vi "Laser_Control_3D.vi"() -> ()   [LabVIEW 2022 SP3]
uses:
  ADAM Client/Sub VIs/ADAM Controls/Update_scan_value.ctl
  Fibre_Flow_Mode.ctl
panel:
  in  "BSA IP Number":string="10.10.100.130"
  in  "Laser3":string="LAN10.10.100.127"
  in  "Laser2":string="LAN10.10.100.121"
  in  "Laser1":string="LAN10.10.100.120"
  out "error out  BSA":errorcluster
  in  "Power (mW) 3":dbl
  out "Status 3":string[](array[string])
  in  "BSALaserCtrl.IBSALaser 4":refnum<k7>
  out "GetMaxPower (mW) 3":dbl
  in  "Mode 3":T1
  out "error out 3":errorcluster
  out "Loop No 3":i32
  in  "Power (mW) 2":dbl
  out "Status 2":string[](array[string])
  in  "BSALaserCtrl.IBSALaser 3":refnum<k7>
  out "GetMaxPower (mW) 2":dbl
  in  "Mode 2":T1
  out "error out 2":errorcluster
  out "Loop No 2":i32
  out "GetMaxPower (mW)":dbl
  in  "stop":bool
  out "Loop No":i32
  in  "Power (mW)":dbl
  in  "Mode":T1
  out "error out":errorcluster
  in  "BSALaserCtrl.IBSALaser 2":refnum<k7>
  out "Status":string[](array[string])
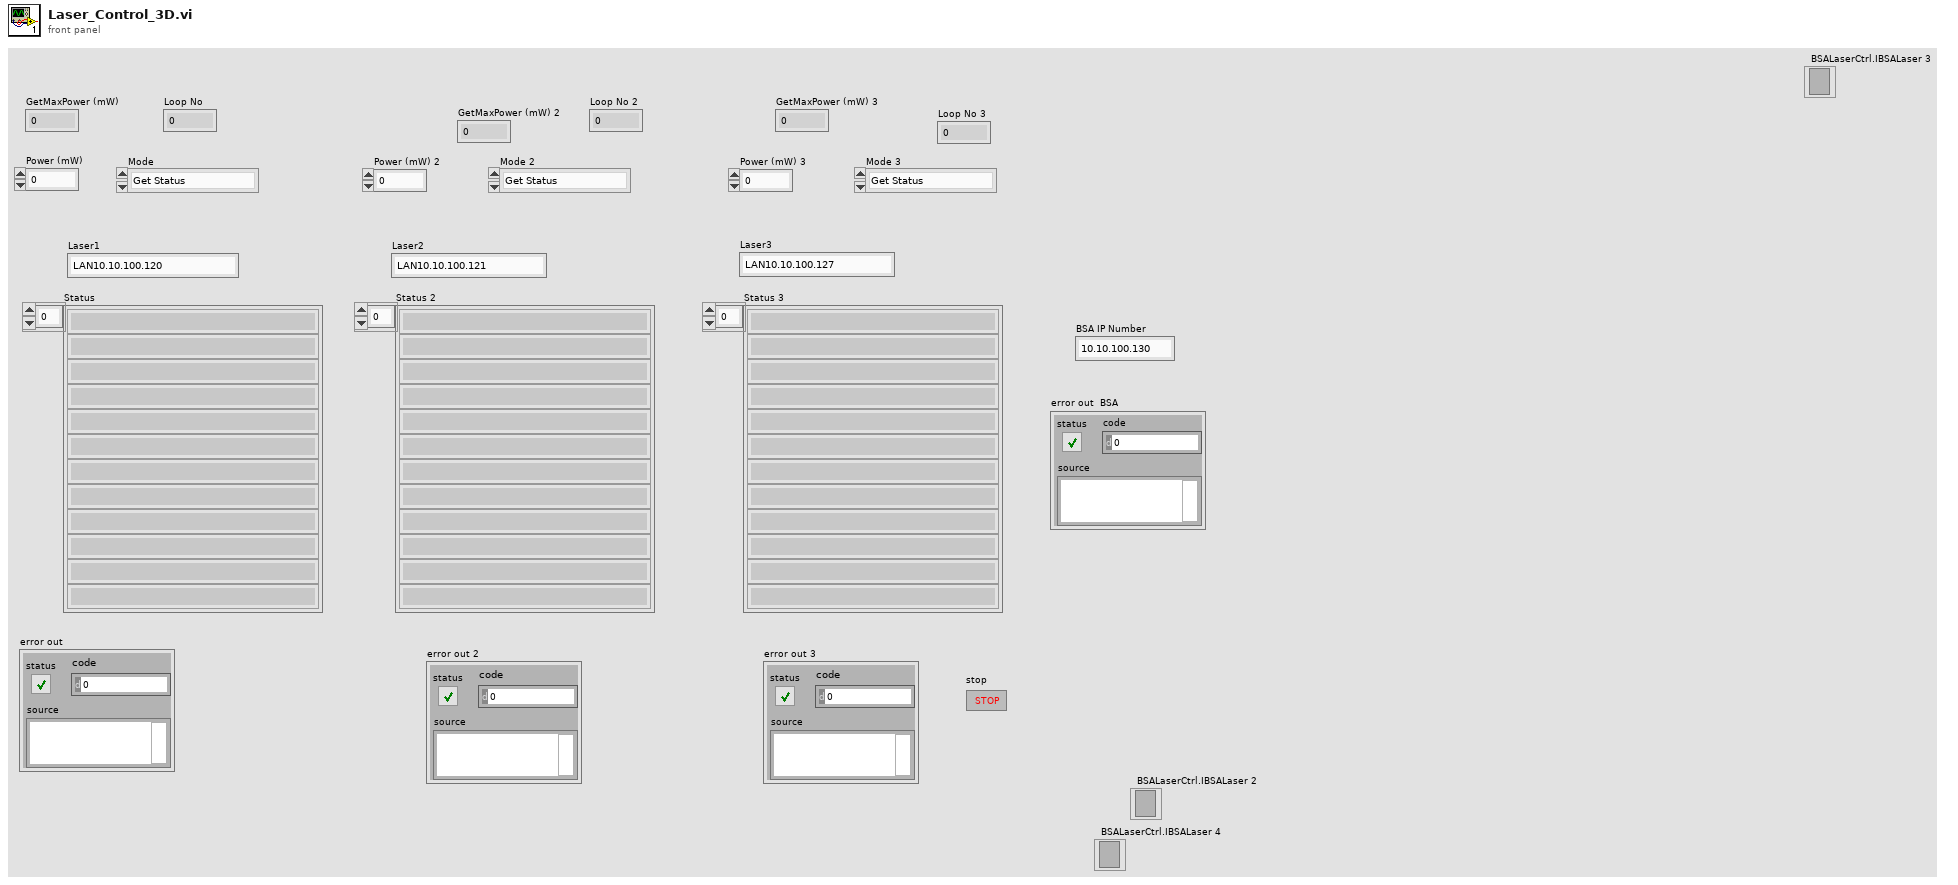
[diagram p1: front panel]
types:
  T1 = typedef "Fibre_Flow_Mode.ctl" = enum16{"Get Status", "Set Power", "Turn Laser On", "Turn Laser Off", "Shutter Open", "Shutter Closed", "Attenuated", "Disconnect"}
  T2 = typedef "Update_scan_value.ctl" = cluster{"Channel Name":string, "New Value":dbl, "!Auto_Off":bool}
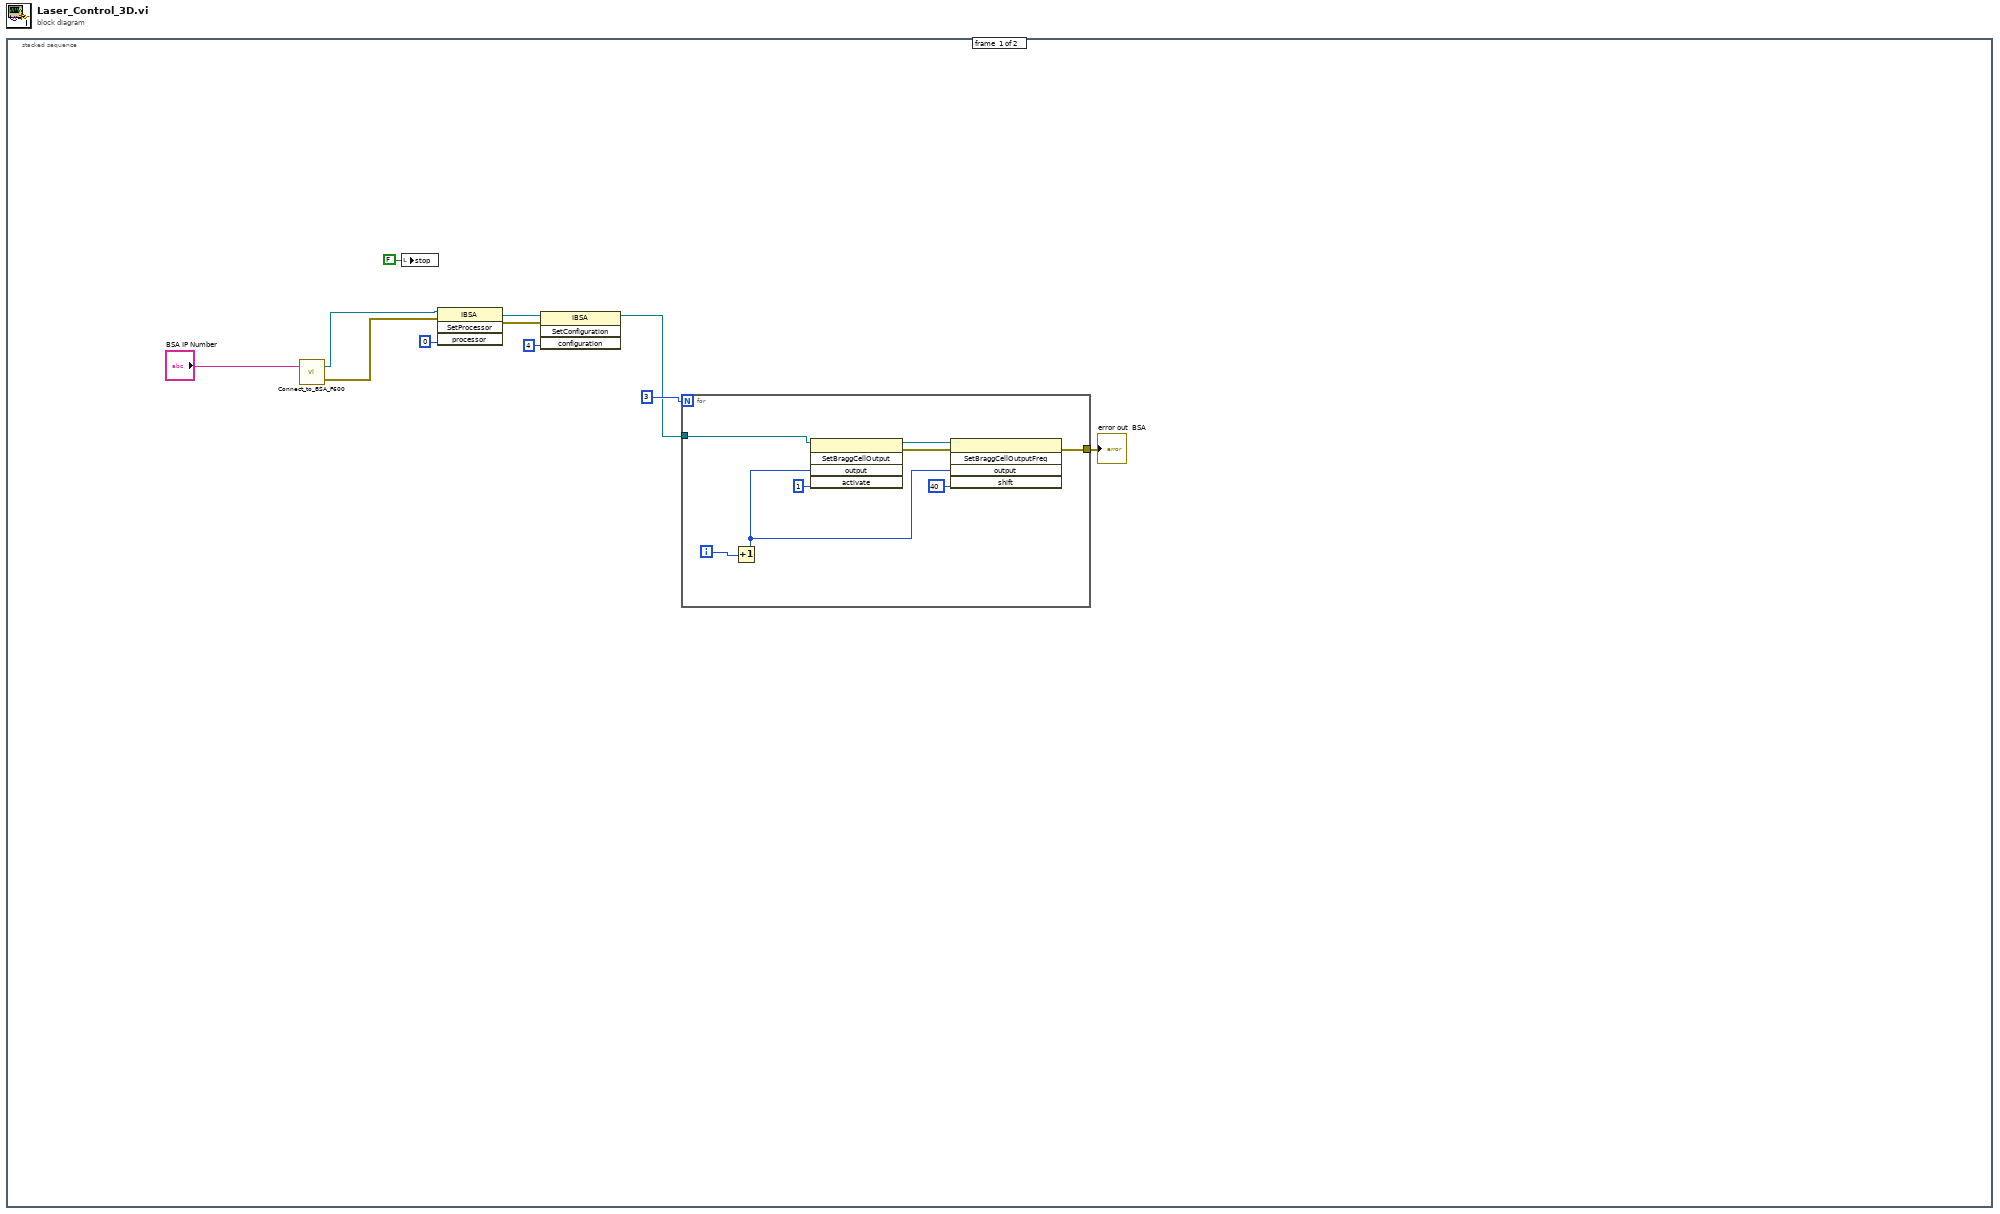
[diagram p0: block diagram]
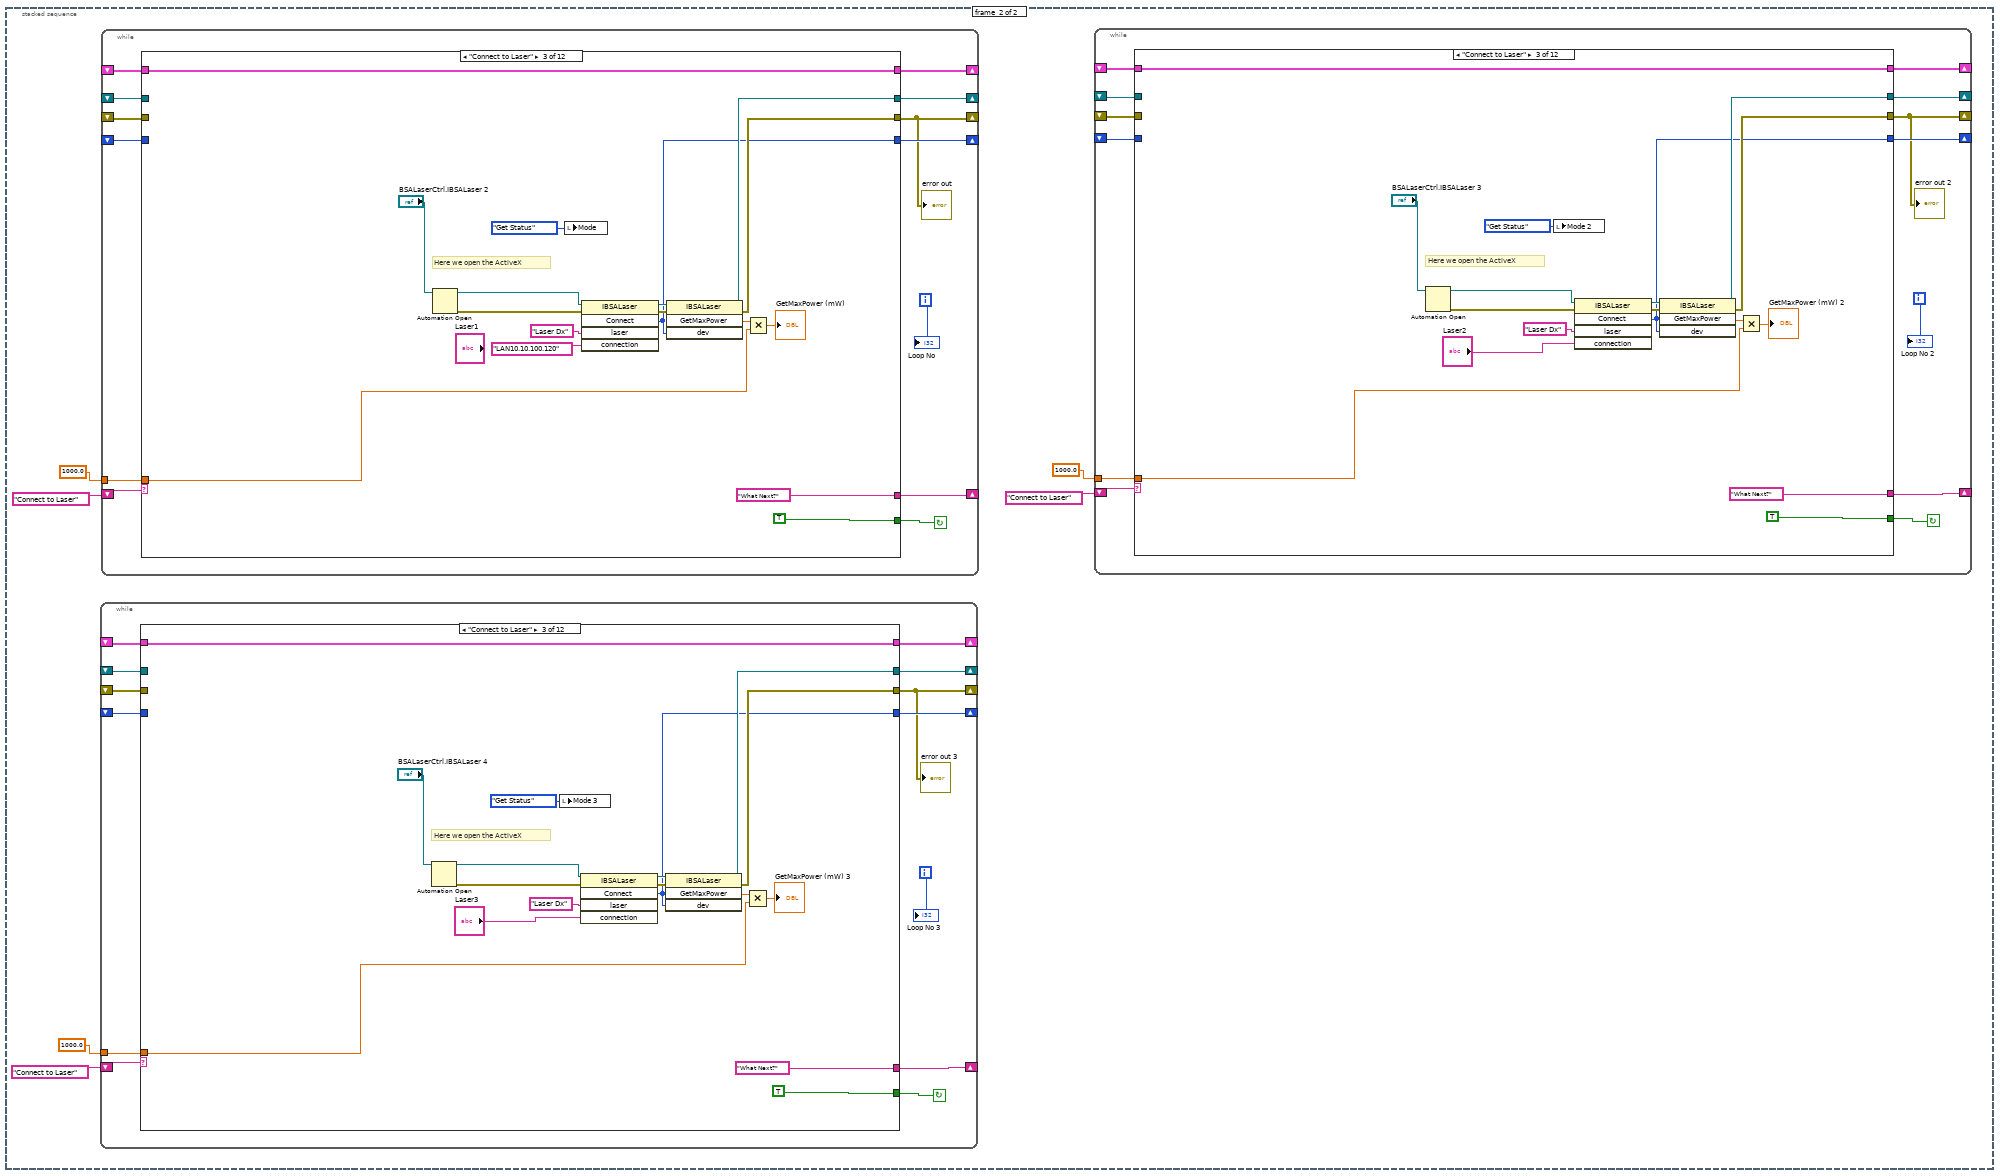
[diagram p2: hidden frame]
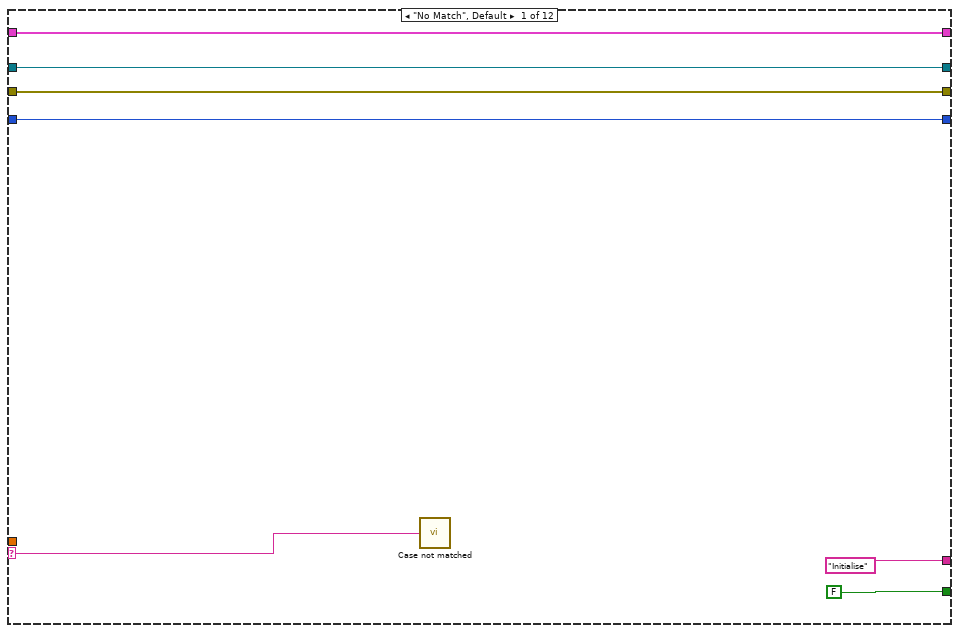
[diagram p3: hidden frame]
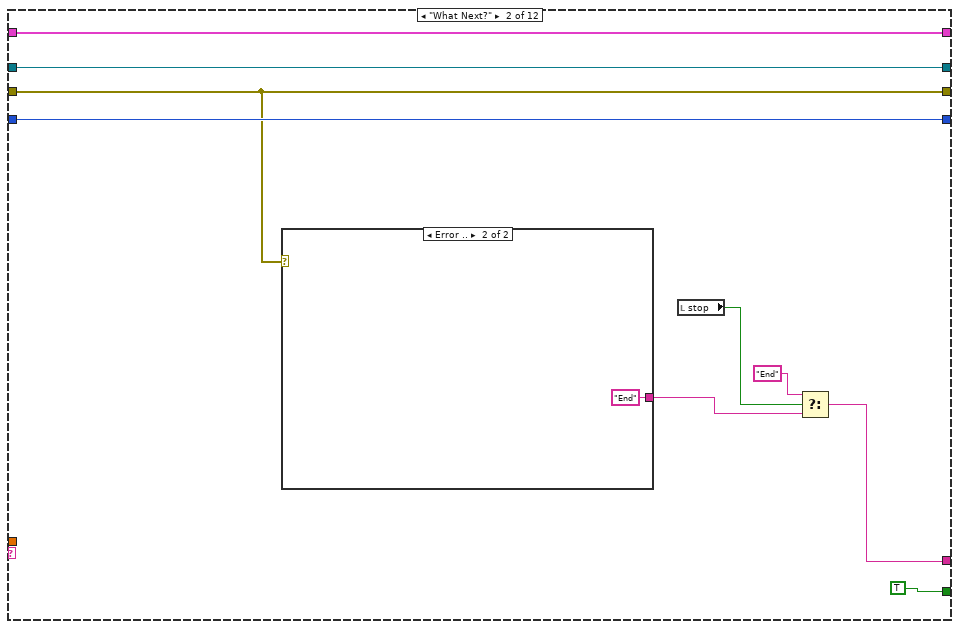
[diagram p4: hidden frame]
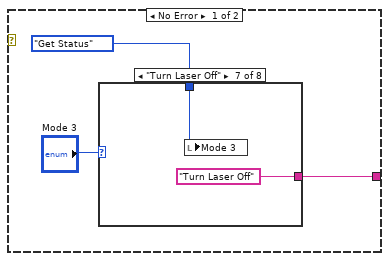
[diagram p5: hidden frame]
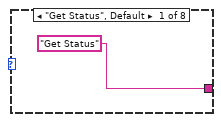
[diagram p6: hidden frame]
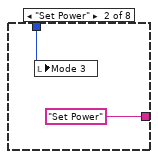
[diagram p7: hidden frame]
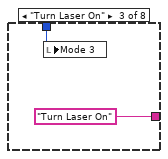
[diagram p8: hidden frame]
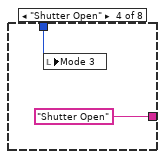
[diagram p9: hidden frame]
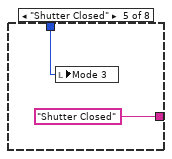
[diagram p10: hidden frame]
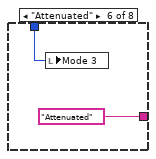
[diagram p11: hidden frame]
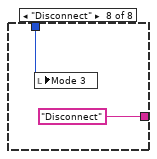
[diagram p12: hidden frame]
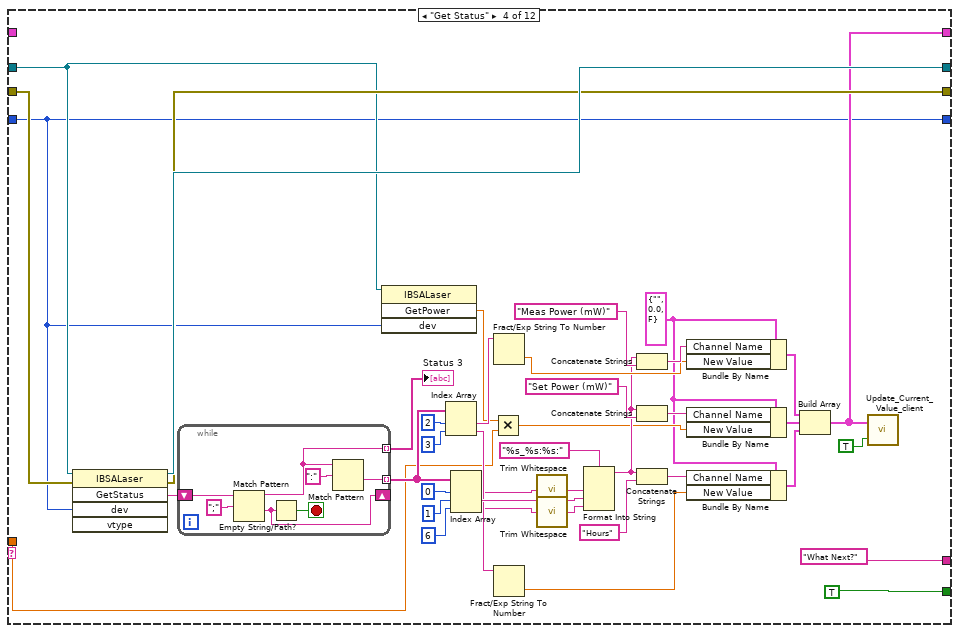
[diagram p13: hidden frame]
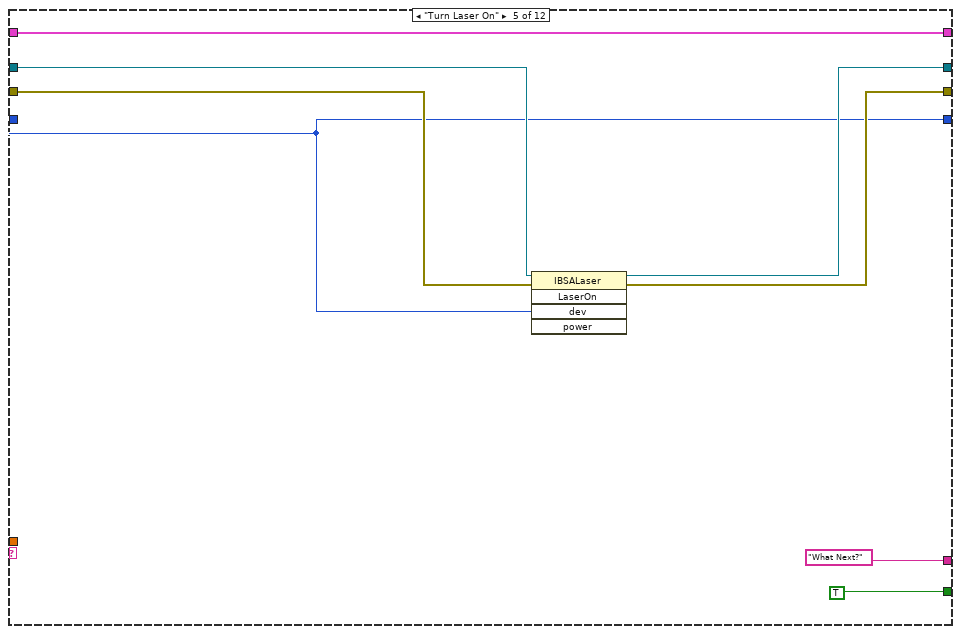
[diagram p14: hidden frame]
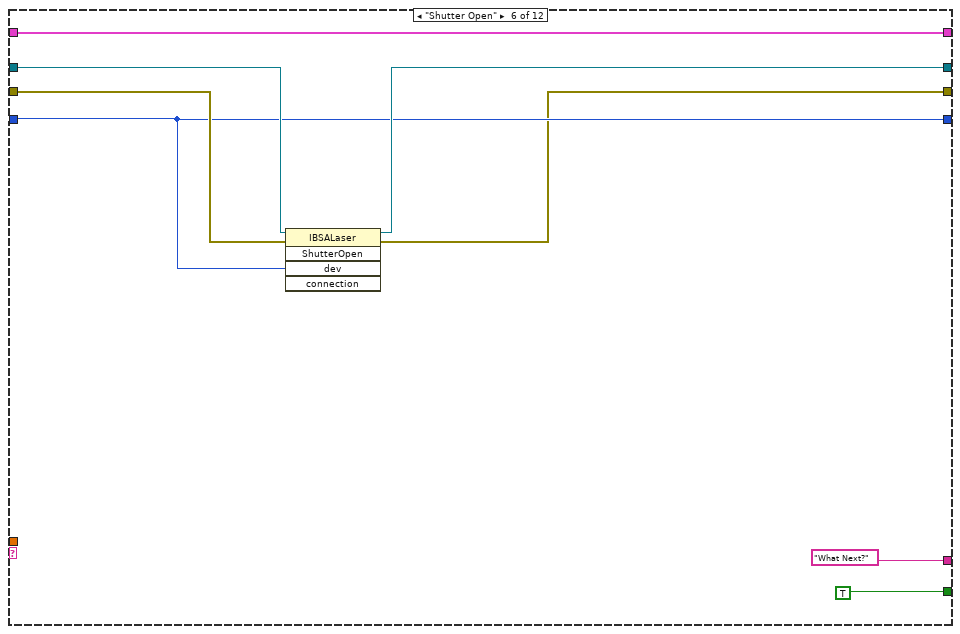
[diagram p15: hidden frame]
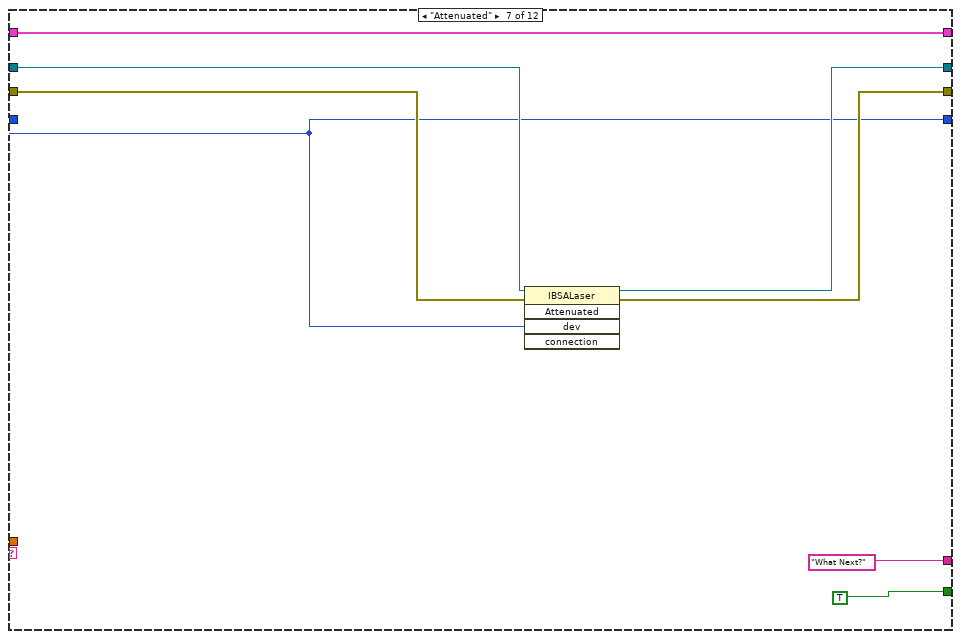
[diagram p16: hidden frame]
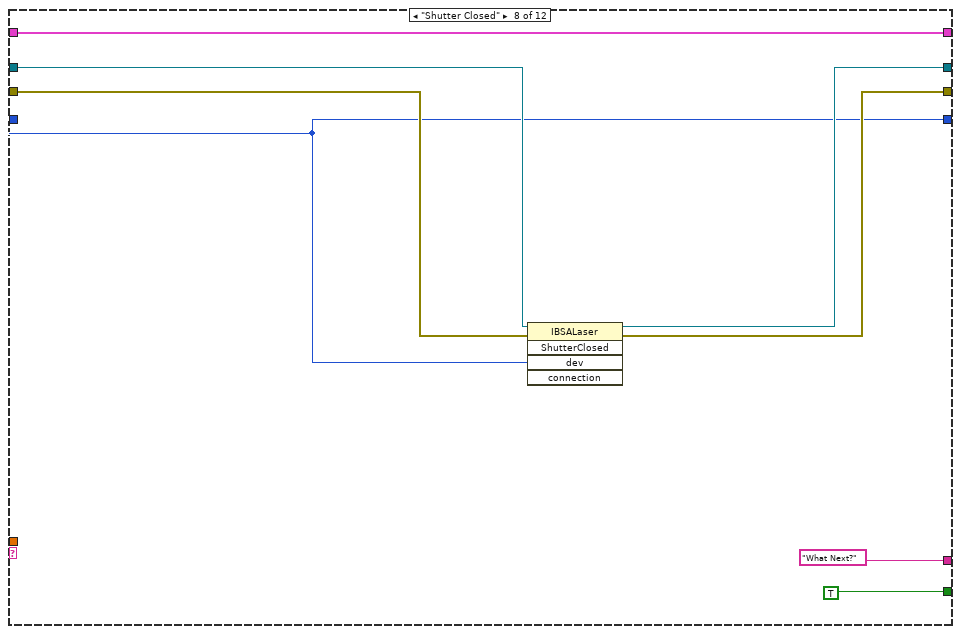
[diagram p17: hidden frame]
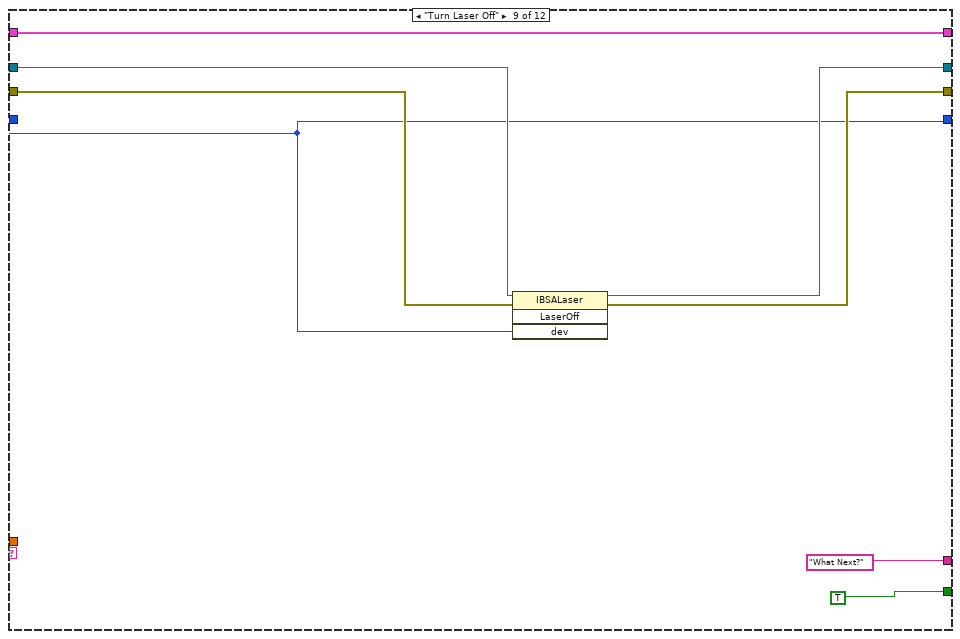
[diagram p18: hidden frame]
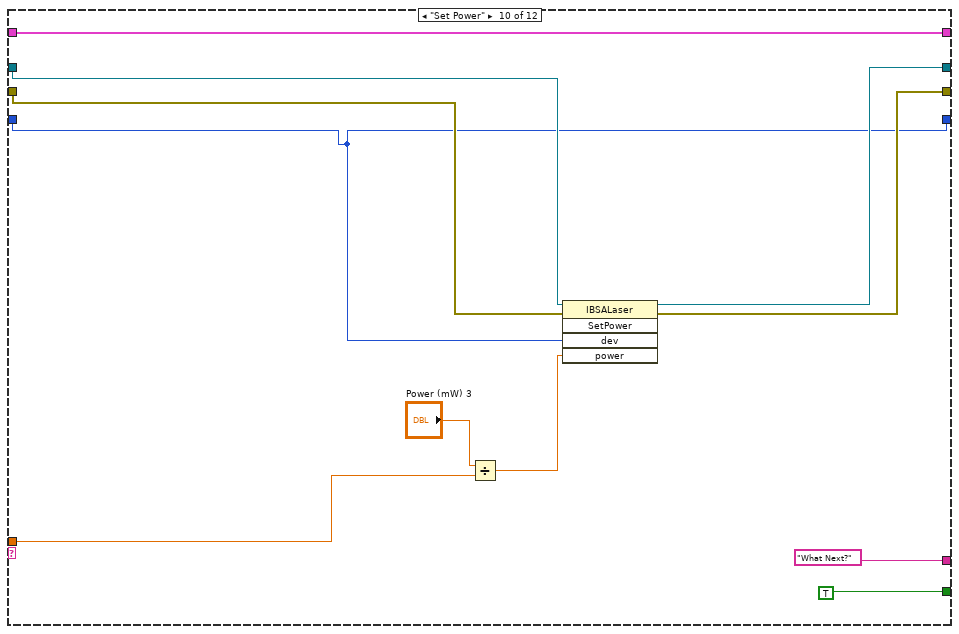
[diagram p19: hidden frame]
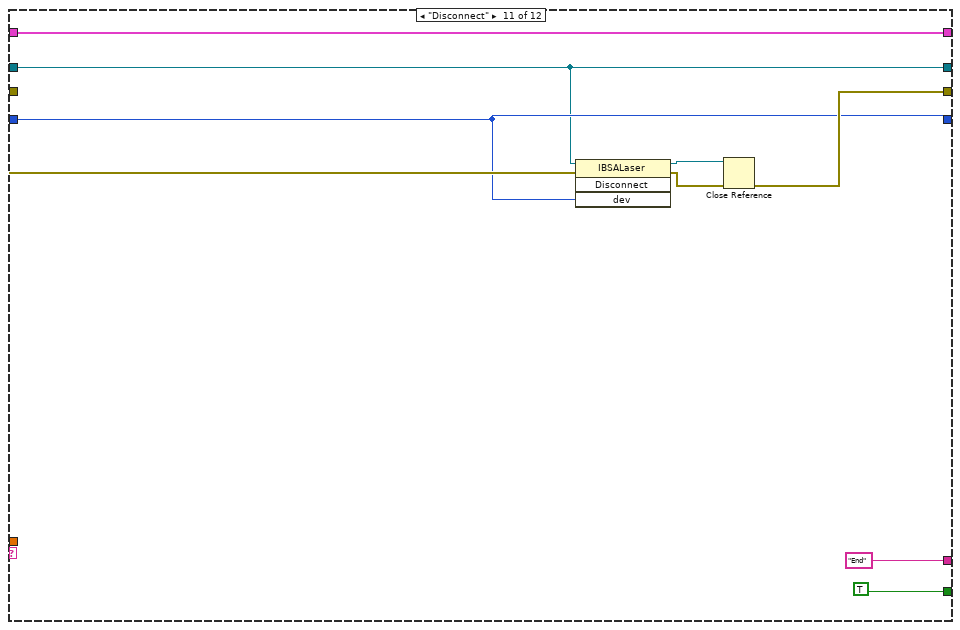
[diagram p20: hidden frame]
diagram:
  n1 = stacked-sequence {
    frame #0 {
      n2 = call "Connect_to_BSA_F600.vi"("BSA IP Number"="BSA IP Number") -> ("error out"=w4:errorcluster, "F600"=w5:refnum<k7>)  [unwired: 1 in]
      n3 = local write "stop"(FALSE ("stop")) -> ()
      n4 = invoke class="IBSA" method="SetProcessor"(reference=w5, error in=w4, "processor"=0) -> (reference out=w7:refnum<k7>, error out=w8:errorcluster)  [unwired: 1 in, 2 out]
      n5 = invoke class="IBSA" method="SetConfiguration"(reference=w7, error in=w8, "configuration"=4) -> (reference out=w3:refnum<k7>)  [unwired: 1 in, 3 out]
      n6 = for {
        N: 3 -> [_]
        tunnel: w3 -> [w15]
        tunnel: [w12] -> w9
        i -> [w14]
        n7 = Increment(x=w14) -> (x+1=w19:i32)
        n8 = invoke method="SetBraggCellOutput"(reference=w15, "output"=w19, "activate"=1) -> (reference out=w17:refnum<k7>, error out=w18:errorcluster)  [unwired: 2 in, 3 out]
        n9 = invoke method="SetBraggCellOutputFreq"(reference=w17, error in=w18, "output"=w19, "shift"=40) -> (error out=w12:errorcluster)  [unwired: 1 in, 4 out]
      }
      "error out  BSA" <- w9
    }
    frame #1 {
      n10 = while {
        shift-left: "Connect to Laser" -> [w36]
        shift-right: [w37] -> _
        shift-right: [w35] -> _
        shift-left: _ -> [w33]
        shift-right: [w30] -> _
        shift-left: _ -> [w32]
        shift-right: [w34] -> _
        shift-left: _ -> [w31]
        shift-right: [w28] -> _
        shift-left: _ -> [w27]
        tunnel: 1000.0 ("y") -> [w26]
        i -> [w29]
        stop <- w38 continue-if-true
        n11 = case shown="\"Connect to Laser\"" w36 {
          selector: w36 -> [w43 _ _ _ _ _ _ _ _ _ _ _]
          tunnel: [FALSE TRUE TRUE TRUE TRUE TRUE TRUE TRUE TRUE TRUE TRUE FALSE] -> w38
          tunnel: ["Initialise" w48 "What Next?" "What Next?" "What Next?" "What Next?" "What Next?" "What Next?" "What Next?" "What Next?" "End" "End"] -> w37
          tunnel: [w42 w54 w81 w127 w142 w150 w158 w166 w174 w185 w191 w203] -> w35
          tunnel: [w41 w52 w80 w126 w141 w147 w157 w165 w173 w184 w193 w202] -> w30
          tunnel: [w40 w53 w79 w101 w140 w149 w156 w164 w172 w183 w192 w204] -> w34
          tunnel: w33 -> [w42 w54 _ w102 w144 w152 w160 w168 w176 w187 w191 w203]
          tunnel: w32 -> [w41 w52 _ w128 w143 w151 w159 w167 w175 w186 w194 w202]
          tunnel: w31 -> [w40 w53 _ w101 w140 w149 w156 w164 w172 w183 w192 w204]
          tunnel: [w39 w51 w84 w103 w139 w148 w155 w163 w171 w182 w190 w200] -> w28
          tunnel: w27 -> [w39 w51 w84 _ w139 w148 w155 w163 w171 w182 w190 w200]
          tunnel: w26 -> [_ _ w76 w94 _ _ _ _ _ w180 _ _]
          frame "No Match", Default {
            n12 = call "Case not matched.vi"("Case Name not Matched"=w43) -> ()
          }
          frame "What Next?" {
            n13 = case shown="Error .." w52 {
              tunnel: [w56 "End"] -> w49
              frame No Error {
                n14 = case shown="\"Turn Laser Off\"" "Mode 3" {
                  tunnel: ["Get Status" "Set Power" "Turn Laser On" "Shutter Open" "Shutter Closed" "Attenuated" "Turn Laser Off" "Disconnect"] -> w56
                  tunnel: Fibre_Flow_Mode."Get Status" ("Mode") -> [_ w59 w61 w63 w65 w67 w69 w71]
                  frame "Get Status", Default {
                  }
                  frame "Set Power" {
                    n15 = local write "Mode 3"(w59) -> ()
                  }
                  frame "Turn Laser On" {
                    n16 = local write "Mode 3"(w61) -> ()
                  }
                  frame "Shutter Open" {
                    n17 = local write "Mode 3"(w63) -> ()
                  }
                  frame "Shutter Closed" {
                    n18 = local write "Mode 3"(w65) -> ()
                  }
                  frame "Attenuated" {
                    n19 = local write "Mode 3"(w67) -> ()
                  }
                  frame "Turn Laser Off" {
                    n20 = local write "Mode 3"(w69) -> ()
                  }
                  frame "Disconnect" {
                    n21 = local write "Mode 3"(w71) -> ()
                  }
                }
              }
              frame Error {
              }
            }
            n22 = local read "stop"() -> (w46:bool)
            n23 = Select(t="End", s=w46, f=w49) -> (s? t:f=w48:string)
          }
          frame "Connect to Laser" {
            # "Here we open the ActiveX"
            n24 = Automation Open(Automation Refnum="BSALaserCtrl.IBSALaser 4") -> (Automation Refnum=w86:refnum<k7>, error out=w87:errorcluster)  [unwired: 3 in]
            n25 = local write "Mode 3"(Fibre_Flow_Mode."Get Status" ("Mode")) -> ()
            n26 = invoke class="IBSALaser" method="Connect"(reference=w86, error in=w87, "laser"="Laser Dx", "connection"="Laser3") -> (reference out=w83:refnum<k7>, error out=w82:errorcluster, "Connect"=w79:i64)  [unwired: 1 in, 2 out]
            n27 = invoke class="IBSALaser" method="GetMaxPower"(reference=w83, error in=w82, "dev"=w79) -> (reference out=w81:refnum<k7>, error out=w80:errorcluster, "GetMaxPower"=w78:dbl)  [unwired: 1 in, 1 out]
            n28 = Multiply(x=w78, y=w76) -> (x*y=→"GetMaxPower (mW) 3":dbl)
          }
          frame "Get Status" {
            w91 = T2 {"Channel Name"="", "New Value"=0.0, "!Auto_Off"=FALSE} ("Update Scan Value Cluster")
            n29 = invoke class="IBSALaser" method="GetStatus"(reference=w102, error in=w128, "dev"=w101) -> (reference out=w127:refnum<k7>, error out=w126:errorcluster, "GetStatus"=w129:string)  [unwired: 2 in, 2 out]
            n30 = while {
              shift-right: [w135] -> _
              shift-left: w129 -> [w137]
              tunnel: [w134] -> w125 mode=indexing
              tunnel: [w132] -> w116 mode=indexing
              stop <- w136 stop-if-true
              n31 = Match Pattern(string=w137, regular expression=";") -> (before substring=w134:string, after substring=w135:string)  [unwired: 1 in, 2 out]
              n32 = Empty String/Path?(string/path=w135) -> (empty?=w136:bool)
              n33 = Match Pattern(string=w134, regular expression=":") -> (after substring=w132:string)  [unwired: 1 in, 3 out]
            }
            "Status 3" <- w125
            n34 = invoke class="IBSALaser" method="GetPower"(reference=w102, "dev"=w101) -> ("GetPower"=w95:dbl)  [unwired: 2 in, 3 out]
            n35 = Index Array(array=w116, index #1=2 ("index"), index #2=3 ("index")) -> (element #1=w113:string, element #2=w111:string)
            n36 = Index Array(array=w116, index #1=0 ("index"), index #2=1 ("index"), index #3=6 ("index")) -> (element #1=w105:string, element #2=w121:string, element #3=w107:string)
            n37 = Multiply(x=w95, y=w94) -> (x*y=w93:dbl)
            n38 = Fract/Exp String To Number(string=w113) -> (number=w112:dbl)  [unwired: 3 in, 1 out]
            n39 = Fract/Exp String To Number(string=w111) -> (number=w98:dbl)  [unwired: 3 in, 1 out]
            n40 = call <vilib>:"Trim Whitespace.vi"("string"=w105) -> ("trimmed string"=w104:string)  [unwired: 1 in]
            n41 = call <vilib>:"Trim Whitespace.vi"("string"=w107) -> ("trimmed string"=w106:string)  [unwired: 1 in]
            n42 = Format Into String(format string="%s_%s:%s:", w104, w121, w106) -> (resulting string=w99:string)  [unwired: 2 in, 1 out]
            n43 = Concatenate Strings(w99, "Meas Power (mW)" ("string")) -> (w117:string)
            n44 = Concatenate Strings(w99, "Set Power (mW)" ("string")) -> (w96:string)
            n45 = Concatenate Strings(w99, "Hours" ("string")) -> (w97:string)
            n46 = Bundle By Name(cluster=w91, "Channel Name"=w117, "New Value"=w112) -> (w110:T2)
            n47 = Bundle By Name(cluster=w91, "Channel Name"=w96, "New Value"=w93) -> (w109:T2)
            n48 = Bundle By Name(cluster=w91, "Channel Name"=w97, "New Value"=w98) -> (w92:T2)
            n49 = Build Array(w110, w109, w92) -> (w103:T2[])
            n50 = call "Update_Current_Value_client.vi"("Don't Bother with check?"=TRUE, "Update array in"=w103) -> ()
          }
          frame "Turn Laser On" {
            n51 = invoke class="IBSALaser" method="LaserOn"(reference=w144, error in=w143, "dev"=w140) -> (reference out=w142:refnum<k7>, error out=w141:errorcluster)  [unwired: 2 in, 3 out]
          }
          frame "Shutter Open" {
            n52 = invoke class="IBSALaser" method="ShutterOpen"(reference=w152, error in=w151, "dev"=w149) -> (reference out=w150:refnum<k7>, error out=w147:errorcluster)  [unwired: 2 in, 3 out]
          }
          frame "Attenuated" {
            n53 = invoke class="IBSALaser" method="Attenuated"(reference=w160, error in=w159, "dev"=w156) -> (reference out=w158:refnum<k7>, error out=w157:errorcluster)  [unwired: 2 in, 3 out]
          }
          frame "Shutter Closed" {
            n54 = invoke class="IBSALaser" method="ShutterClosed"(reference=w168, error in=w167, "dev"=w164) -> (reference out=w166:refnum<k7>, error out=w165:errorcluster)  [unwired: 2 in, 3 out]
          }
          frame "Turn Laser Off" {
            n55 = invoke class="IBSALaser" method="LaserOff"(reference=w176, error in=w175, "dev"=w172) -> (reference out=w174:refnum<k7>, error out=w173:errorcluster)  [unwired: 1 in, 2 out]
          }
          frame "Set Power" {
            n56 = Divide(x="Power (mW) 3", y=w180) -> (x/y=w179:dbl)
            n57 = invoke class="IBSALaser" method="SetPower"(reference=w187, error in=w186, "dev"=w183, "power"=w179) -> (reference out=w185:refnum<k7>, error out=w184:errorcluster)  [unwired: 1 in, 3 out]
          }
          frame "Disconnect" {
            n58 = invoke class="IBSALaser" method="Disconnect"(reference=w191, error in=w194, "dev"=w192) -> (reference out=w195:refnum<k7>, error out=w196:errorcluster)  [unwired: 1 in, 2 out]
            n59 = Close Reference(reference=w195, error in (no error)=w196) -> (error out=w193:errorcluster)
          }
          frame "End" {
            n60 = for {
              tunnel: [w208] -> w199 mode=indexing
              tunnel: w200 -> [w207] mode=indexing
              n61 = Bundle By Name(cluster=w207, "New Value"=nan) -> (w208:T2)
            }
            n62 = call "Update_Current_Value_client.vi"("Don't Bother with check?"=TRUE, "Update array in"=w199) -> ()
          }
        }
        "error out 3" <- w30
        "Loop No 3" <- w29
      }
      n63 = while {
        shift-left: "Connect to Laser" -> [w404]
        shift-right: [w405] -> _
        shift-right: [w403] -> _
        shift-left: _ -> [w401]
        shift-right: [w398] -> _
        shift-left: _ -> [w400]
        shift-right: [w402] -> _
        shift-left: _ -> [w399]
        shift-right: [w396] -> _
        shift-left: _ -> [w395]
        tunnel: 1000.0 ("y") -> [w394]
        i -> [w397]
        stop <- w406 continue-if-true
        n64 = case shown="\"Connect to Laser\"" w404 {
          selector: w404 -> [w411 _ _ _ _ _ _ _ _ _ _ _]
          tunnel: [FALSE TRUE TRUE TRUE TRUE TRUE TRUE TRUE TRUE TRUE TRUE FALSE] -> w406
          tunnel: ["Initialise" w415 "What Next?" "What Next?" "What Next?" "What Next?" "What Next?" "What Next?" "What Next?" "What Next?" "End" "End"] -> w405
          tunnel: [w410 w422 w448 w495 w510 w518 w526 w534 w542 w553 w559 w571] -> w403
          tunnel: [w409 w420 w447 w494 w509 w515 w525 w533 w541 w552 w561 w570] -> w398
          tunnel: [w408 w421 w446 w469 w508 w517 w524 w532 w540 w551 w560 w572] -> w402
          tunnel: w401 -> [w410 w422 _ w470 w512 w520 w528 w536 w544 w555 w559 w571]
          tunnel: w400 -> [w409 w420 _ w496 w511 w519 w527 w535 w543 w554 w562 w570]
          tunnel: w399 -> [w408 w421 _ w469 w508 w517 w524 w532 w540 w551 w560 w572]
          tunnel: [w407 w419 w451 w471 w507 w516 w523 w531 w539 w550 w558 w568] -> w396
          tunnel: w395 -> [w407 w419 w451 _ w507 w516 w523 w531 w539 w550 w558 w568]
          tunnel: w394 -> [_ _ w443 w462 _ _ _ _ _ w548 _ _]
          frame "No Match", Default {
            n65 = call "Case not matched.vi"("Case Name not Matched"=w411) -> ()
          }
          frame "What Next?" {
            n66 = case shown="Error .." w420 {
              tunnel: [w424 "End"] -> w416
              frame No Error {
                n67 = case shown="\"Disconnect\"" "Mode" {
                  tunnel: ["Get Status" "Set Power" "Turn Laser On" "Shutter Open" "Shutter Closed" "Attenuated" "Turn Laser Off" "Disconnect"] -> w424
                  tunnel: Fibre_Flow_Mode."Get Status" ("Mode") -> [_ w427 w429 w431 w433 w435 w437 w439]
                  frame "Get Status", Default {
                  }
                  frame "Set Power" {
                    n68 = local write "Mode"(w427) -> ()
                  }
                  frame "Turn Laser On" {
                    n69 = local write "Mode"(w429) -> ()
                  }
                  frame "Shutter Open" {
                    n70 = local write "Mode"(w431) -> ()
                  }
                  frame "Shutter Closed" {
                    n71 = local write "Mode"(w433) -> ()
                  }
                  frame "Attenuated" {
                    n72 = local write "Mode"(w435) -> ()
                  }
                  frame "Turn Laser Off" {
                    n73 = local write "Mode"(w437) -> ()
                  }
                  frame "Disconnect" {
                    n74 = local write "Mode"(w439) -> ()
                  }
                }
              }
              frame Error {
              }
            }
            n75 = Select(t="End", s="stop", f=w416) -> (s? t:f=w415:string)
          }
          frame "Connect to Laser" {
            # "Here we open the ActiveX"
            n76 = Automation Open(Automation Refnum="BSALaserCtrl.IBSALaser 2") -> (Automation Refnum=w454:refnum<k7>, error out=w455:errorcluster)  [unwired: 3 in]
            n77 = local write "Mode"(Fibre_Flow_Mode."Get Status" ("Mode")) -> ()
            n78 = invoke class="IBSALaser" method="Connect"(reference=w454, error in=w455, "laser"="Laser Dx", "connection"="LAN10.10.100.120") -> (reference out=w450:refnum<k7>, error out=w449:errorcluster, "Connect"=w446:i64)  [unwired: 1 in, 2 out]
            n79 = invoke class="IBSALaser" method="GetMaxPower"(reference=w450, error in=w449, "dev"=w446) -> (reference out=w448:refnum<k7>, error out=w447:errorcluster, "GetMaxPower"=w445:dbl)  [unwired: 1 in, 1 out]
            n80 = Multiply(x=w445, y=w443) -> (x*y=→"GetMaxPower (mW)":dbl)
          }
          frame "Get Status" {
            w459 = T2 {"Channel Name"="", "New Value"=0.0, "!Auto_Off"=FALSE} ("Update Scan Value Cluster")
            n81 = invoke class="IBSALaser" method="GetStatus"(reference=w470, error in=w496, "dev"=w469) -> (reference out=w495:refnum<k7>, error out=w494:errorcluster, "GetStatus"=w497:string)  [unwired: 2 in, 2 out]
            n82 = while {
              shift-right: [w503] -> _
              shift-left: w497 -> [w505]
              tunnel: [w502] -> w493 mode=indexing
              tunnel: [w500] -> w484 mode=indexing
              stop <- w504 stop-if-true
              n83 = Match Pattern(string=w505, regular expression=";") -> (before substring=w502:string, after substring=w503:string)  [unwired: 1 in, 2 out]
              n84 = Empty String/Path?(string/path=w503) -> (empty?=w504:bool)
              n85 = Match Pattern(string=w502, regular expression=":") -> (after substring=w500:string)  [unwired: 1 in, 3 out]
            }
            "Status" <- w493
            n86 = invoke class="IBSALaser" method="GetPower"(reference=w470, "dev"=w469) -> ("GetPower"=w463:dbl)  [unwired: 2 in, 3 out]
            n87 = Index Array(array=w484, index #1=2 ("index"), index #2=3 ("index")) -> (element #1=w481:string, element #2=w479:string)
            n88 = Index Array(array=w484, index #1=0 ("index"), index #2=1 ("index"), index #3=6 ("index")) -> (element #1=w473:string, element #2=w489:string, element #3=w475:string)
            n89 = Multiply(x=w463, y=w462) -> (x*y=w461:dbl)
            n90 = Fract/Exp String To Number(string=w481) -> (number=w480:dbl)  [unwired: 3 in, 1 out]
            n91 = Fract/Exp String To Number(string=w479) -> (number=w466:dbl)  [unwired: 3 in, 1 out]
            n92 = call <vilib>:"Trim Whitespace.vi"("string"=w473) -> ("trimmed string"=w472:string)  [unwired: 1 in]
            n93 = call <vilib>:"Trim Whitespace.vi"("string"=w475) -> ("trimmed string"=w474:string)  [unwired: 1 in]
            n94 = Format Into String(format string="%s_%s:%s:", w472, w489, w474) -> (resulting string=w467:string)  [unwired: 2 in, 1 out]
            n95 = Concatenate Strings(w467, "Meas Power (mW)" ("string")) -> (w485:string)
            n96 = Concatenate Strings(w467, "Set Power (mW)" ("string")) -> (w464:string)
            n97 = Concatenate Strings(w467, "Hours" ("string")) -> (w465:string)
            n98 = Bundle By Name(cluster=w459, "Channel Name"=w485, "New Value"=w480) -> (w478:T2)
            n99 = Bundle By Name(cluster=w459, "Channel Name"=w464, "New Value"=w461) -> (w477:T2)
            n100 = Bundle By Name(cluster=w459, "Channel Name"=w465, "New Value"=w466) -> (w460:T2)
            n101 = Build Array(w478, w477, w460) -> (w471:T2[])
            n102 = call "Update_Current_Value_client.vi"("Don't Bother with check?"=TRUE, "Update array in"=w471) -> ()
          }
          frame "Turn Laser On" {
            n103 = invoke class="IBSALaser" method="LaserOn"(reference=w512, error in=w511, "dev"=w508) -> (reference out=w510:refnum<k7>, error out=w509:errorcluster)  [unwired: 2 in, 3 out]
          }
          frame "Shutter Open" {
            n104 = invoke class="IBSALaser" method="ShutterOpen"(reference=w520, error in=w519, "dev"=w517) -> (reference out=w518:refnum<k7>, error out=w515:errorcluster)  [unwired: 2 in, 3 out]
          }
          frame "Attenuated" {
            n105 = invoke class="IBSALaser" method="Attenuated"(reference=w528, error in=w527, "dev"=w524) -> (reference out=w526:refnum<k7>, error out=w525:errorcluster)  [unwired: 2 in, 3 out]
          }
          frame "Shutter Closed" {
            n106 = invoke class="IBSALaser" method="ShutterClosed"(reference=w536, error in=w535, "dev"=w532) -> (reference out=w534:refnum<k7>, error out=w533:errorcluster)  [unwired: 2 in, 3 out]
          }
          frame "Turn Laser Off" {
            n107 = invoke class="IBSALaser" method="LaserOff"(reference=w544, error in=w543, "dev"=w540) -> (reference out=w542:refnum<k7>, error out=w541:errorcluster)  [unwired: 1 in, 2 out]
          }
          frame "Set Power" {
            n108 = Divide(x="Power (mW)", y=w548) -> (x/y=w547:dbl)
            n109 = invoke class="IBSALaser" method="SetPower"(reference=w555, error in=w554, "dev"=w551, "power"=w547) -> (reference out=w553:refnum<k7>, error out=w552:errorcluster)  [unwired: 1 in, 3 out]
          }
          frame "Disconnect" {
            n110 = invoke class="IBSALaser" method="Disconnect"(reference=w559, error in=w562, "dev"=w560) -> (reference out=w563:refnum<k7>, error out=w564:errorcluster)  [unwired: 1 in, 2 out]
            n111 = Close Reference(reference=w563, error in (no error)=w564) -> (error out=w561:errorcluster)
          }
          frame "End" {
            n112 = for {
              tunnel: [w576] -> w567 mode=indexing
              tunnel: w568 -> [w575] mode=indexing
              n113 = Bundle By Name(cluster=w575, "New Value"=nan) -> (w576:T2)
            }
            n114 = call "Update_Current_Value_client.vi"("Don't Bother with check?"=TRUE, "Update array in"=w567) -> ()
          }
        }
        "error out" <- w398
        "Loop No" <- w397
      }
      n115 = while {
        shift-left: "Connect to Laser" -> [w220]
        shift-right: [w221] -> _
        shift-right: [w219] -> _
        shift-left: _ -> [w217]
        shift-right: [w214] -> _
        shift-left: _ -> [w216]
        shift-right: [w218] -> _
        shift-left: _ -> [w215]
        shift-right: [w212] -> _
        shift-left: _ -> [w211]
        tunnel: 1000.0 ("y") -> [w210]
        i -> [w213]
        stop <- w222 continue-if-true
        n116 = case shown="\"Connect to Laser\"" w220 {
          selector: w220 -> [w227 _ _ _ _ _ _ _ _ _ _ _]
          tunnel: [FALSE TRUE TRUE TRUE TRUE TRUE TRUE TRUE TRUE TRUE TRUE FALSE] -> w222
          tunnel: ["Initialise" w232 "What Next?" "What Next?" "What Next?" "What Next?" "What Next?" "What Next?" "What Next?" "What Next?" "End" "End"] -> w221
          tunnel: [w226 w238 w265 w311 w326 w334 w342 w350 w358 w369 w375 w387] -> w219
          tunnel: [w225 w236 w264 w310 w325 w331 w341 w349 w357 w368 w377 w386] -> w214
          tunnel: [w224 w237 w263 w285 w324 w333 w340 w348 w356 w367 w376 w388] -> w218
          tunnel: w217 -> [w226 w238 _ w286 w328 w336 w344 w352 w360 w371 w375 w387]
          tunnel: w216 -> [w225 w236 _ w312 w327 w335 w343 w351 w359 w370 w378 w386]
          tunnel: w215 -> [w224 w237 _ w285 w324 w333 w340 w348 w356 w367 w376 w388]
          tunnel: [w223 w235 w268 w287 w323 w332 w339 w347 w355 w366 w374 w384] -> w212
          tunnel: w211 -> [w223 w235 w268 _ w323 w332 w339 w347 w355 w366 w374 w384]
          tunnel: w210 -> [_ _ w260 w278 _ _ _ _ _ w364 _ _]
          frame "No Match", Default {
            n117 = call "Case not matched.vi"("Case Name not Matched"=w227) -> ()
          }
          frame "What Next?" {
            n118 = case shown="Error .." w236 {
              tunnel: [w240 "End"] -> w233
              frame No Error {
                n119 = case shown="\"Turn Laser Off\"" "Mode 2" {
                  tunnel: ["Get Status" "Set Power" "Turn Laser On" "Shutter Open" "Shutter Closed" "Attenuated" "Turn Laser Off" "Disconnect"] -> w240
                  tunnel: Fibre_Flow_Mode."Get Status" ("Mode") -> [_ w243 w245 w247 w249 w251 w253 w255]
                  frame "Get Status", Default {
                  }
                  frame "Set Power" {
                    n120 = local write "Mode 2"(w243) -> ()
                  }
                  frame "Turn Laser On" {
                    n121 = local write "Mode 2"(w245) -> ()
                  }
                  frame "Shutter Open" {
                    n122 = local write "Mode 2"(w247) -> ()
                  }
                  frame "Shutter Closed" {
                    n123 = local write "Mode 2"(w249) -> ()
                  }
                  frame "Attenuated" {
                    n124 = local write "Mode 2"(w251) -> ()
                  }
                  frame "Turn Laser Off" {
                    n125 = local write "Mode 2"(w253) -> ()
                  }
                  frame "Disconnect" {
                    n126 = local write "Mode 2"(w255) -> ()
                  }
                }
              }
              frame Error {
              }
            }
            n127 = local read "stop"() -> (w230:bool)
            n128 = Select(t="End", s=w230, f=w233) -> (s? t:f=w232:string)
          }
          frame "Connect to Laser" {
            # "Here we open the ActiveX"
            n129 = Automation Open(Automation Refnum="BSALaserCtrl.IBSALaser 3") -> (Automation Refnum=w270:refnum<k7>, error out=w271:errorcluster)  [unwired: 3 in]
            n130 = local write "Mode 2"(Fibre_Flow_Mode."Get Status" ("Mode")) -> ()
            n131 = invoke class="IBSALaser" method="Connect"(reference=w270, error in=w271, "laser"="Laser Dx", "connection"="Laser2") -> (reference out=w267:refnum<k7>, error out=w266:errorcluster, "Connect"=w263:i64)  [unwired: 1 in, 2 out]
            n132 = invoke class="IBSALaser" method="GetMaxPower"(reference=w267, error in=w266, "dev"=w263) -> (reference out=w265:refnum<k7>, error out=w264:errorcluster, "GetMaxPower"=w262:dbl)  [unwired: 1 in, 1 out]
            n133 = Multiply(x=w262, y=w260) -> (x*y=→"GetMaxPower (mW) 2":dbl)
          }
          frame "Get Status" {
            w275 = T2 {"Channel Name"="", "New Value"=0.0, "!Auto_Off"=FALSE} ("Update Scan Value Cluster")
            n134 = invoke class="IBSALaser" method="GetStatus"(reference=w286, error in=w312, "dev"=w285) -> (reference out=w311:refnum<k7>, error out=w310:errorcluster, "GetStatus"=w313:string)  [unwired: 2 in, 2 out]
            n135 = while {
              shift-right: [w319] -> _
              shift-left: w313 -> [w321]
              tunnel: [w318] -> w309 mode=indexing
              tunnel: [w316] -> w300 mode=indexing
              stop <- w320 stop-if-true
              n136 = Match Pattern(string=w321, regular expression=";") -> (before substring=w318:string, after substring=w319:string)  [unwired: 1 in, 2 out]
              n137 = Empty String/Path?(string/path=w319) -> (empty?=w320:bool)
              n138 = Match Pattern(string=w318, regular expression=":") -> (after substring=w316:string)  [unwired: 1 in, 3 out]
            }
            "Status 2" <- w309
            n139 = invoke class="IBSALaser" method="GetPower"(reference=w286, "dev"=w285) -> ("GetPower"=w279:dbl)  [unwired: 2 in, 3 out]
            n140 = Index Array(array=w300, index #1=2 ("index"), index #2=3 ("index")) -> (element #1=w297:string, element #2=w295:string)
            n141 = Index Array(array=w300, index #1=0 ("index"), index #2=1 ("index"), index #3=6 ("index")) -> (element #1=w289:string, element #2=w305:string, element #3=w291:string)
            n142 = Multiply(x=w279, y=w278) -> (x*y=w277:dbl)
            n143 = Fract/Exp String To Number(string=w297) -> (number=w296:dbl)  [unwired: 3 in, 1 out]
            n144 = Fract/Exp String To Number(string=w295) -> (number=w282:dbl)  [unwired: 3 in, 1 out]
            n145 = call <vilib>:"Trim Whitespace.vi"("string"=w289) -> ("trimmed string"=w288:string)  [unwired: 1 in]
            n146 = call <vilib>:"Trim Whitespace.vi"("string"=w291) -> ("trimmed string"=w290:string)  [unwired: 1 in]
            n147 = Format Into String(format string="%s_%s:%s:", w288, w305, w290) -> (resulting string=w283:string)  [unwired: 2 in, 1 out]
            n148 = Concatenate Strings(w283, "Meas Power (mW)" ("string")) -> (w301:string)
            n149 = Concatenate Strings(w283, "Set Power (mW)" ("string")) -> (w280:string)
            n150 = Concatenate Strings(w283, "Hours" ("string")) -> (w281:string)
            n151 = Bundle By Name(cluster=w275, "Channel Name"=w301, "New Value"=w296) -> (w294:T2)
            n152 = Bundle By Name(cluster=w275, "Channel Name"=w280, "New Value"=w277) -> (w293:T2)
            n153 = Bundle By Name(cluster=w275, "Channel Name"=w281, "New Value"=w282) -> (w276:T2)
            n154 = Build Array(w294, w293, w276) -> (w287:T2[])
            n155 = call "Update_Current_Value_client.vi"("Don't Bother with check?"=TRUE, "Update array in"=w287) -> ()
          }
          frame "Turn Laser On" {
            n156 = invoke class="IBSALaser" method="LaserOn"(reference=w328, error in=w327, "dev"=w324) -> (reference out=w326:refnum<k7>, error out=w325:errorcluster)  [unwired: 2 in, 3 out]
          }
          frame "Shutter Open" {
            n157 = invoke class="IBSALaser" method="ShutterOpen"(reference=w336, error in=w335, "dev"=w333) -> (reference out=w334:refnum<k7>, error out=w331:errorcluster)  [unwired: 2 in, 3 out]
          }
          frame "Attenuated" {
            n158 = invoke class="IBSALaser" method="Attenuated"(reference=w344, error in=w343, "dev"=w340) -> (reference out=w342:refnum<k7>, error out=w341:errorcluster)  [unwired: 2 in, 3 out]
          }
          frame "Shutter Closed" {
            n159 = invoke class="IBSALaser" method="ShutterClosed"(reference=w352, error in=w351, "dev"=w348) -> (reference out=w350:refnum<k7>, error out=w349:errorcluster)  [unwired: 2 in, 3 out]
          }
          frame "Turn Laser Off" {
            n160 = invoke class="IBSALaser" method="LaserOff"(reference=w360, error in=w359, "dev"=w356) -> (reference out=w358:refnum<k7>, error out=w357:errorcluster)  [unwired: 1 in, 2 out]
          }
          frame "Set Power" {
            n161 = Divide(x="Power (mW) 2", y=w364) -> (x/y=w363:dbl)
            n162 = invoke class="IBSALaser" method="SetPower"(reference=w371, error in=w370, "dev"=w367, "power"=w363) -> (reference out=w369:refnum<k7>, error out=w368:errorcluster)  [unwired: 1 in, 3 out]
          }
          frame "Disconnect" {
            n163 = invoke class="IBSALaser" method="Disconnect"(reference=w375, error in=w378, "dev"=w376) -> (reference out=w379:refnum<k7>, error out=w380:errorcluster)  [unwired: 1 in, 2 out]
            n164 = Close Reference(reference=w379, error in (no error)=w380) -> (error out=w377:errorcluster)
          }
          frame "End" {
            n165 = for {
              tunnel: [w392] -> w383 mode=indexing
              tunnel: w384 -> [w391] mode=indexing
              n166 = Bundle By Name(cluster=w391, "New Value"=nan) -> (w392:T2)
            }
            n167 = call "Update_Current_Value_client.vi"("Don't Bother with check?"=TRUE, "Update array in"=w383) -> ()
          }
        }
        "error out 2" <- w214
        "Loop No 2" <- w213
      }
    }
  }
